vi "coordsTaker.vi"(8 "image data":T2, 11 "coords":cluster{dbl, dbl, dbl, dbl}) -> (3 "Cluster out":T1)   [LabVIEW 2020]
uses:
  <vilib>/picture/picture.llb/imagedata.ctl
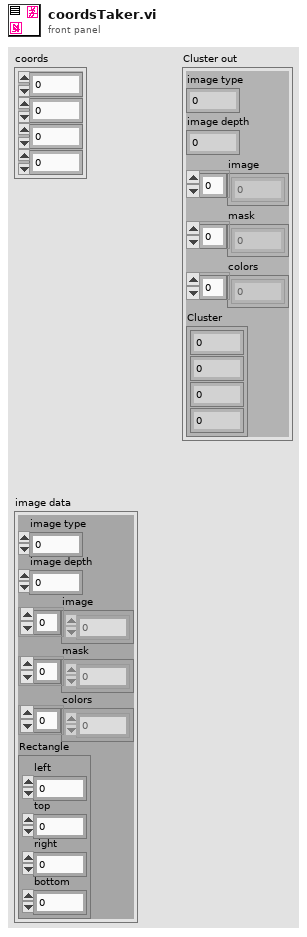
[diagram p1: front panel]
types:
  T1 = cluster{"image type":i32, "image depth":i32, "image":u8[], "mask":u8[], "colors":u32[], "Cluster":cluster{dbl, dbl, dbl, dbl}}
  T2 = typedef "imagedata.ctl" = cluster{"image type":i32, "image depth":i32, "image":u8[], "mask":u8[], "colors":u32[], "Rectangle":cluster{"left":i16, "top":i16, "right":i16, "bottom":i16}}
  T3 = cluster{"image type":i32, "image depth":i32, "image":u8[], "mask":u8[], "colors":u32[], "coords":cluster{dbl, dbl, dbl, dbl}}
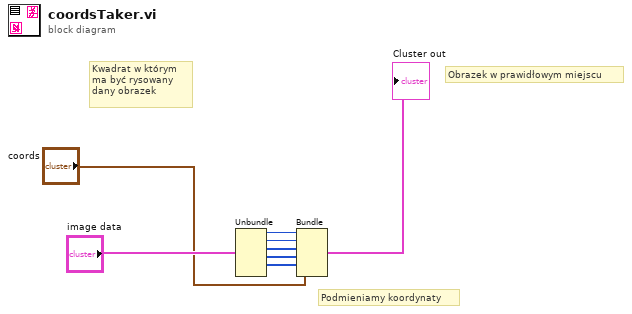
[diagram p0: block diagram]
diagram:
  # "Obrazek w prawidłowym miejscu"
  # "Podmieniamy koordynaty"
  # "Kwadrat w którym ma być rysowany dany obrazek"
  n1 = Unbundle("image data") -> ("image type"=w1:i32, "image depth"=w8:i32, "image"=w2:u8[], "mask"=w3:u8[], "colors"=w4:u32[])  [unwired: 1 out]
  n2 = Bundle("image type"=w1, "image depth"=w8, "image"=w2, "mask"=w3, "colors"=w4, "coords"="coords") -> (→"Cluster out":T3)  [unwired: 1 in]
